vi "ReadState.vi"(8 "Error In":errorcluster, 11 "Queue In":refnum<queue>) -> (0 "Error Out":errorcluster, 1 "Data":variant, 2 "State":string, 3 "Queue Out":refnum<queue>)   [LabVIEW 2010]
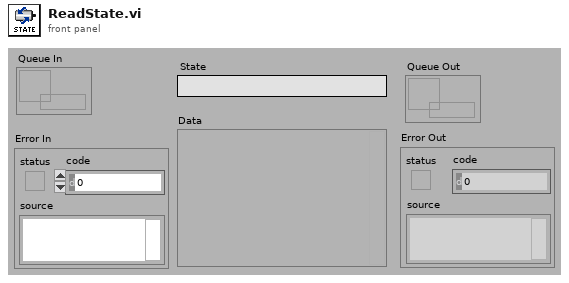
[diagram p1: front panel]
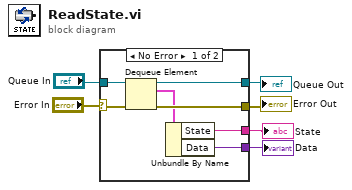
[diagram p0: block diagram]
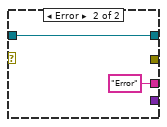
[diagram p2: hidden frame]
diagram:
  n1 = case shown="No Error" "Error In" {
    selector: "Error In" -> [w13 _]
    tunnel: [w12 _] -> w5
    tunnel: [w11 w15] -> w4
    tunnel: "Queue In" -> [w10 w15]
    tunnel: [w8 "Error" ("State")] -> w2
    tunnel: [w7 _] -> w1
    frame No Error {
      n2 = Dequeue Element(queue=w10, error in (no error)=w13) -> (queue out=w11:refnum<queue>, element=w9:cluster{"State":string, "Data":variant}, error out=w12:errorcluster)  [unwired: 1 in, 1 out]
      n3 = Unbundle By Name(w9) -> ("State"=w8:string, "Data"=w7:variant)
    }
    frame Error {
    }
  }
  "Data" <- w1
  "State" <- w2
  "Queue Out" <- w4
  "Error Out" <- w5
